vi "Send to Single Connection.vi"(7 "Connection ID":string, 8 "error in (no error)":errorcluster, 9 "Data":variant, 10 "Message":string, 11 "Multiplexed Messenger In":refnum<data-value>) -> (0 "error out":errorcluster, 3 "Multiplexed Messenger Out":refnum<data-value>)   [LabVIEW 2020, in "Network Messenger.lvlib" / "Multiplexed Messenger.lvclass"]
uses:
  <vilib>/gpm_packages/@cs/Network-interface/Source/Network Messenger/Multiplexed Messenger/Multiplexed Messenger.lvclass
  <vilib>/gpm_packages/@cs/Network-interface/Source/Network Messenger/Multiplexed Messenger/Multiplexed Messenger.lvclass/Multiplexed Messenger.ctl
  <vilib>/gpm_packages/@cs/Network-interface/Source/Network Messenger/Synchronous Write Callback/Synchronous Write Callback.lvclass/Synchronous Write Callback.ctl
  <vilib>/gpm_packages/@cs/Network-interface/Source/Network Messenger/Types/Message Packet.ctl
  <vilib>/gpm_packages/@cs/Network-interface/Source/MessagingInterfaces/WriteRequest/WriteRequest.lvclass/WriteRequest.ctl
  <vilib>/gpm_packages/@cs/Network-interface/Source/MultiplexedConnectionHandler/MultiplexedConnectionHandler Messages/Execute Single Point Write Request Msg/Execute Single Point Write Request Msg.lvclass/Execute Single Point Write Request Msg.ctl
  <vilib>/ActorFramework/Message Enqueuer/Message Enqueuer.lvclass/Message Enqueuer.ctl
  <vilib>/ActorFramework/Message Enqueuer/Enqueue.vi
  <vilib>/gpm_packages/@cs/Network-interface/Source/Network Messenger/Synchronous Write Callback/Synchronous Write Callback.lvclass
  C:/Program Files/National Instruments/LabVIEW 2020/vi.lib/gpm_packages/@cs/Network-interface/Source/MessagingInterfaces/IWriteExecutionCallback/IWriteExecutionCallback.lvclass
  <vilib>/gpm_packages/@cs/Network-interface/Source/Network Messenger/ClusterMessagePacket/ClusterMessagePacket.lvclass
  C:/Program Files/National Instruments/LabVIEW 2020/vi.lib/gpm_packages/@cs/Network-interface/Source/MessagingInterfaces/IPacket/IPacket.lvclass
  <vilib>/gpm_packages/@cs/Network-interface/Source/MultiplexedConnectionHandler/MultiplexedConnectionHandler Messages/Execute Single Point Write Request Msg/Execute Single Point Write Request Msg.lvclass
  C:/Program Files/National Instruments/LabVIEW 2020/vi.lib/ActorFramework/Message/Message.lvclass
  <vilib>/ActorFramework/Message Priority Queue/Priority Enqueue.vi
  <vilib>/gpm_packages/@cs/Network-interface/Source/MessagingInterfaces/WriteRequest/WriteRequest.lvclass
  <vilib>/gpm_packages/@cs/Network-interface/Source/Network Messenger/Network Messenger.lvlib
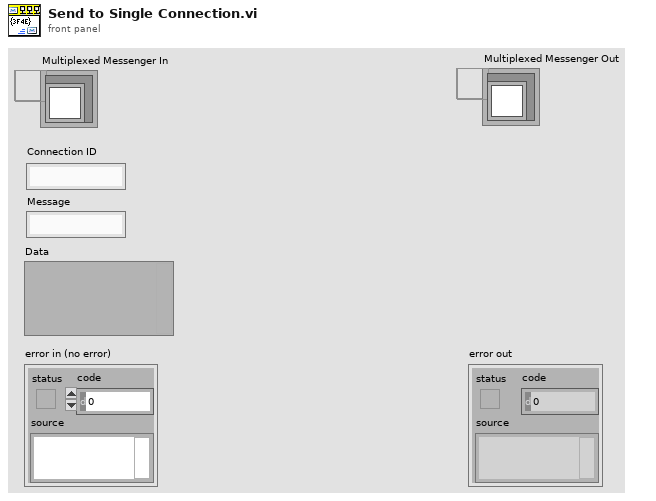
[diagram p1: front panel]
types:
  T1 = typedef "Network Messenger.lvlib/Message Packet.ctl" = cluster{"Msg":string, "Data":variant}
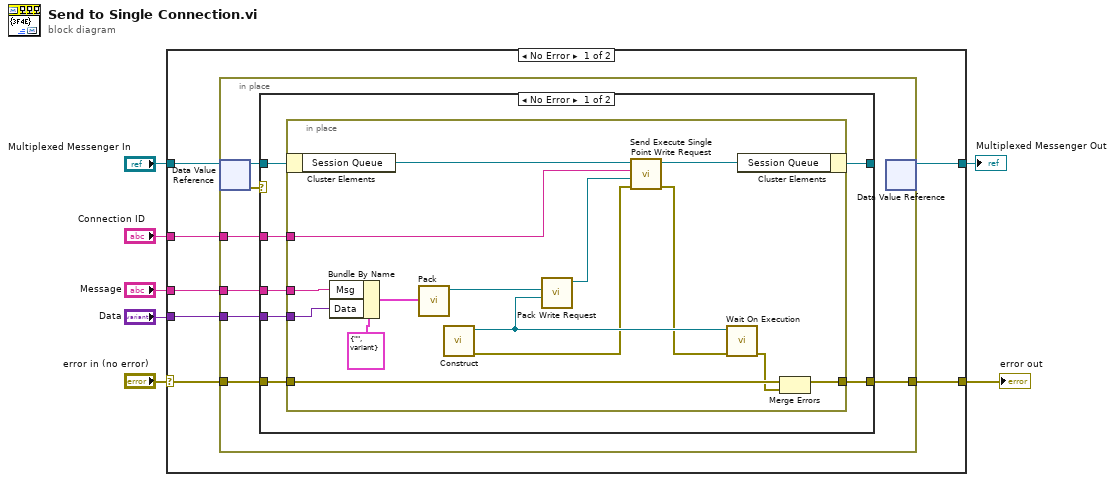
[diagram p0: block diagram]
diagram:
  n1 = case shown="No Error" "error in (no error)" {
    selector: "error in (no error)" -> [w12 w46]
    tunnel: "Multiplexed Messenger In" -> [w14 w47]
    tunnel: [w13 w47] -> w4
    tunnel: "Message" -> [w11 _]
    tunnel: "Data" -> [w10 _]
    tunnel: [w9 w46] -> w7
    tunnel: "Connection ID" -> [w8 _]
    frame No Error {
      n2 = in-place {
        in-place-border: w12 -> [w19]
        in-place-border: w11 -> [w17]
        in-place-border: w10 -> [w16]
        in-place-border: [w18] -> w9
        in-place-border: w8 -> [w15]
        n3 = in-place-dvr #1(w14) -> (w21:refnum<class "Multiplexed Messenger.lvclass">, w20:errorcluster)
        n4 = case shown="No Error" w20 {
          selector: w20 -> [_ w44]
          tunnel: w21 -> [w28 w45]
          tunnel: [w27 w45] -> _
          tunnel: w19 -> [w26 _]
          tunnel: [w25 w44] -> w18
          tunnel: w17 -> [w24 _]
          tunnel: w16 -> [w23 _]
          tunnel: w15 -> [w22 _]
          frame No Error {
            n5 = in-place {
              in-place-border: w26 -> [w43]
              in-place-border: [w37] -> w25
              in-place-border: w24 -> [w40]
              in-place-border: w23 -> [w39]
              in-place-border: w22 -> [w29]
              n6 = in-place-cluster #2(w28) -> ("Session Queue"=w34:refnum<class "Message Enqueuer.lvclass">)
              n7 = Bundle By Name(cluster=T1 {"Msg"="", "Data"=variant} ("Packet"), "Msg"=w40, "Data"=w39) -> (w41:T1)
              n8 = call <vilib>:"Pack.vi"("Packet"=w41) -> ("ClusterMessagePacket out"=w38:refnum<class "ClusterMessagePacket.lvclass">)  [unwired: 10 in]
              n9 = call <vilib>:"Construct.vi"() -> ("error out"=w32:errorcluster, "SynchronousWriteCallback out"=w35:refnum<class "Synchronous Write Callback.lvclass">)  [unwired: 10 in]
              n10 = call <vilib>:"Pack Write Request.vi"("Execution Callback"=w35, "Packet"=w38) -> ("WriteRequest out"=w30:refnum<class "WriteRequest.lvclass">)  [unwired: 9 in]
              n11 = call <vilib>:"Send Execute Single Point Write Request.vi"("error in (no error)"=w32, "Write Request"=w30, "Connection ID"=w29, "Message Enqueuer"=w34) -> ("error out"=w31:errorcluster, "Message Enqueuer out"=w33:refnum<class "Message Enqueuer.lvclass">)  [unwired: 6 in]
              n12 = call <vilib>:"Wait On Execution.vi"("error in (no error)"=w31, "Synchronous Write Callback in"=w35) -> ("error out"=w36:errorcluster)  [unwired: 9 in]
              n13 = in-place-cluster #2("Session Queue"=w33) -> (w27:refnum<class "Multiplexed Messenger.lvclass">)
              n14 = Merge Errors(w43, w36) -> (w37:errorcluster)
            }
          }
          frame Error {
          }
        }
        n15 = in-place-dvr #1() -> (w13:refnum<data-value>)  [unwired: 1 in, 1 out]
      }
    }
    frame Error {
    }
  }
  "error out" <- w7
  "Multiplexed Messenger Out" <- w4
